vi "GlobalVI.vi"() -> ()   [LabVIEW 2016]
doc: "Global variables for the Unicorn Main"
panel:
  out "subscriberStatus":bool
  out "publisherStatus":bool
  out "error out":errorcluster
  in  "FPGA VI Reference":refnum<k20>
  out "ledState":i32
  out "activeLed":i32
  out "robotDirection":i32
  out "unicornState":i32
  out "avgDist":sgl
  out "currentLiftState":i32
  out "lightStatus":bool
  out "uwbStatus":bool
  out "lidarBackStatus":bool
  out "liftStatus":bool
  out "emergencyStop":bool
  out "runLidarBack":bool
  in  "position":cluster{"x":dbl, "y":dbl, "z":dbl}
  out "runLiftStatemachine":bool
  # "Lift Statemachine"
  # "R2100 Lidar"
  # "UWB Position"
  # "System Status"
  # "LED Strip"
  # "ROS"
  # "FPGA"
  # "DO NOT TOUCH"
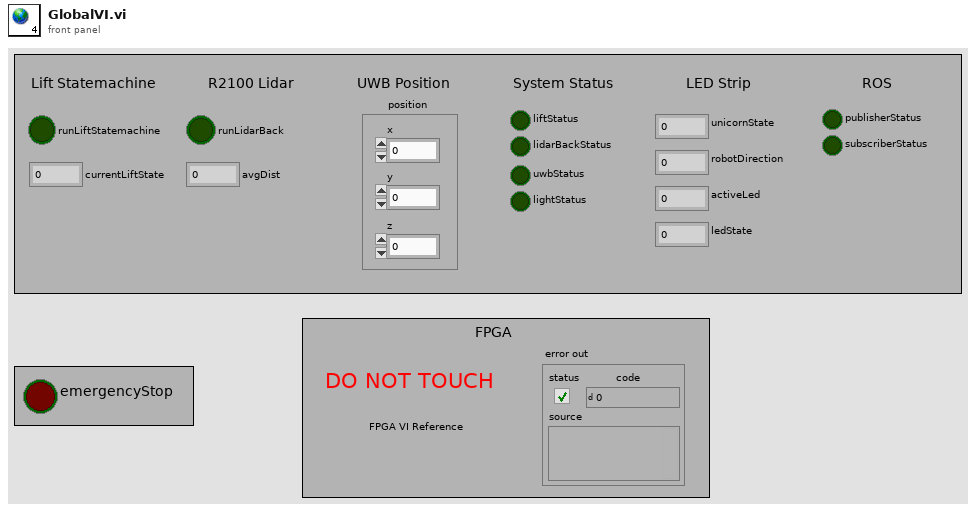
[diagram p1: front panel]
diagram:
